vi "Stop or Cancel Analog Out.vi"(9 "Stop":bool, 10 "Cancel":bool, 11 "ADALM2000 Handler":u32 caption="Instrument Handle Out") -> (3 "ADALM2000 Handler 2":u32 caption="Instrument Handle Out")   [LabVIEW 2015]
uses:
  libm2k_lv.dll
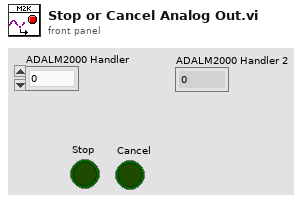
[diagram p1: front panel]
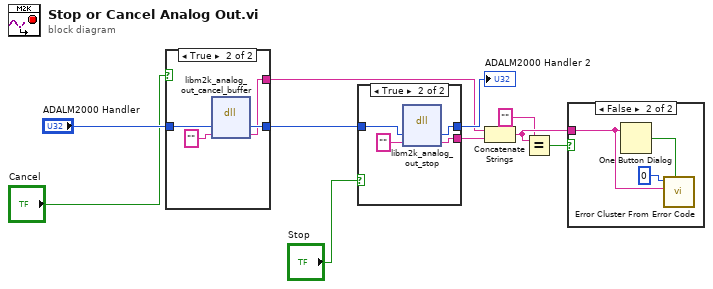
[diagram p0: block diagram]
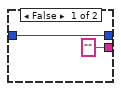
[diagram p3: hidden frame]
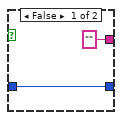
[diagram p4: hidden frame]
diagram:
  n1 = case shown="True" "Cancel" {
    tunnel: "ADALM2000 Handler" -> [w12 w16]
    tunnel: [w12 w15] -> w9
    tunnel: ["" ("err") w13] -> w7
    frame False {
    }
    frame True {
      n2 = dll-call lib="libm2k_lv.*" fn="libm2k_analog_out_cancel_buffer"("instance"=w16, "err"="") -> ("instance"=w15:u64, "err"=w13:string)  [unwired: 4 in, 2 out]
    }
  }
  n3 = case shown="True" "Stop" {
    tunnel: w9 -> [w18 w22]
    tunnel: [w18 w21] -> w8
    tunnel: ["" ("err") w20] -> w6
    frame False {
    }
    frame True {
      n4 = dll-call lib="libm2k_lv.*" fn="libm2k_analog_out_stop"("instance"=w22, "err"="") -> ("instance"=w21:u64, "err"=w20:string)  [unwired: 4 in, 2 out]
    }
  }
  "ADALM2000 Handler 2" <- w8
  n5 = Concatenate Strings(w7, w6) -> (w4:string)
  n6 = Equal?(x=w4, y="") -> (x = y?=w5:bool)
  n7 = case shown="False" w5 {
    tunnel: w4 -> [_ w23]
    frame True {
    }
    frame False {
      n8 = One Button Dialog(message=w23) -> (true=w25:bool)  [unwired: 1 in]
      n9 = call <vilib>:"Error Cluster From Error Code.vi"("show call chain? (False)"=w25, "error message (\"\")"=w23, "error code (0)"=0) -> ()  [unwired: 6 in, 1 out]
    }
  }
